vi "Protocol.Filter by Device Address.vi"(8 "error in":errorcluster, 10 "CAN Frame":T5 {"payload" format="%x"; "timestamp" format="%<%.7X\n%x>T"; "type" items=["CAN Data"=0, "CAN Remote"=1, "CAN Bus Error"=2, "CAN 2.0 Data"=8, "CAN FD Data"=16, "CAN FD+BRS Data"=24, "J1939 Data"=192, "Delay"=224, "Log Trigger"=225, "Start Trigger"=226]; "identifier" format="%x"}, 11 "J1939 Cluster":T2) -> (0 "error out":errorcluster, 1 "Pass Through":bool, 3 "State":T1=enum."ACL")   [LabVIEW 2023, in "J1939 Addon Engine.lvlib"]
uses:
  J1939 Addon Engine.lvlib
  <vilib>/xnet/xnet.llb/XNET Frame CAN.ctl
  <vilib>/xnet/xnet.llb/XNET Frame Type CAN.ctl
  Types/Protocol.Refs.ctl
  Support Libraries/J1939 Utilities/Types/CAN Outgoing Message Cluster.ctl
  Types/Protocol.RQST Lookup Table Reference.ctl
  Types/Protocol.Address Table Reference.ctl
  Support Libraries/J1939 Utilities/Types/Message Types.ctl
  Support Libraries/J1939 Utilities/J1939 Utilities.lvlib
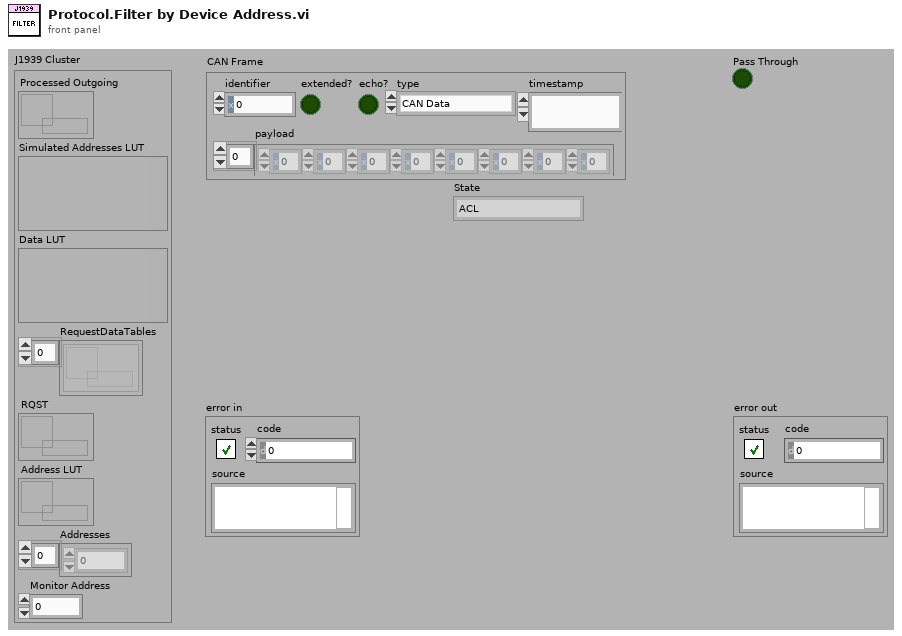
[diagram p1: front panel]
types:
  T1 = typedef "J1939 Utilities.lvlib/Message Types.ctl" = enum8{"PDU 1", "RQST2", "XFER", "ACKM", "RQST", "TP.DT - RTS/CTS", "TP.DT - BAM", "TP.CM - RTS", "TP.CM - CTS", "TP.CM - EndofMsgACK", "TP.CM - BAM", "TP.CM - Abort", "TP.CM - Error", "ACL", "Proprietary A", "PDU 2", "Proprietary B", "Error"}
  T2 = typedef "J1939 Addon Engine.lvlib/Protocol.Refs.ctl" = cluster{"Processed Outgoing":refnum<queue>, "Simulated Addresses LUT":variant, "Data LUT":variant, "RequestDataTables":refnum<k33>[], "RQST":T3, "Address LUT":T4, "Addresses":u8[], "Monitor Address":u8}
  T3 = typedef "J1939 Addon Engine.lvlib/Protocol.RQST Lookup Table Reference.ctl" = refnum<data-value>
  T4 = typedef "J1939 Addon Engine.lvlib/Protocol.Address Table Reference.ctl" = refnum<data-value>
  T5 = typedef "XNET Frame CAN.ctl" = cluster{"timestamp":timestamp, "payload":u8[], "identifier":u32, "type":T6, "extended?":bool, "echo?":bool}
  T6 = typedef "XNET Frame Type CAN.ctl" = u8
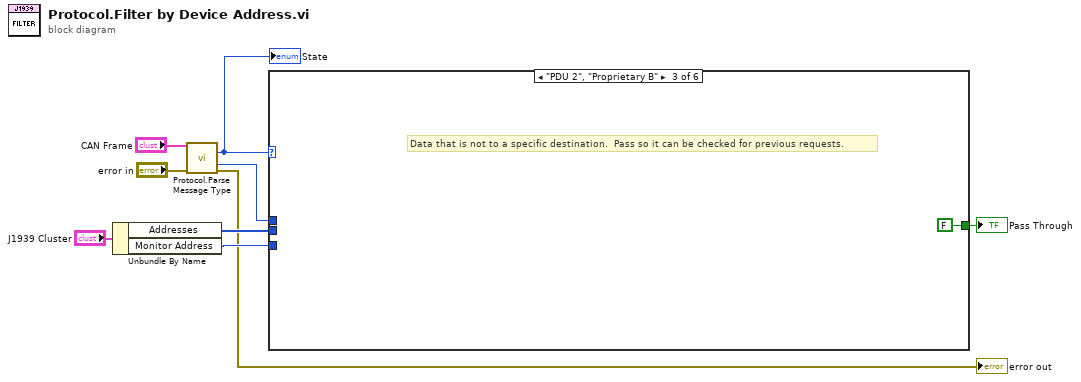
[diagram p0: block diagram]
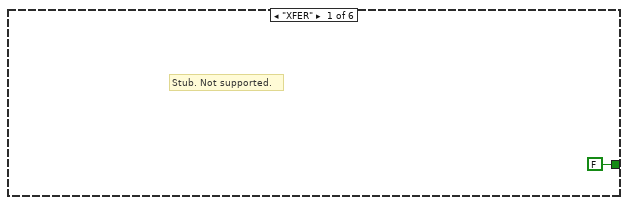
[diagram p2: hidden frame]
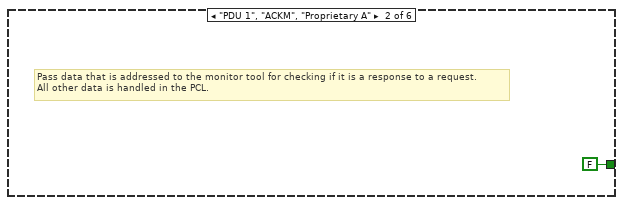
[diagram p3: hidden frame]
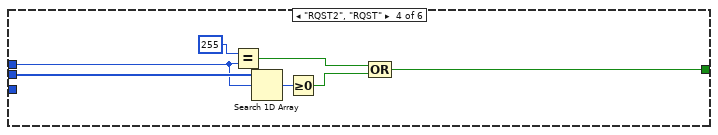
[diagram p4: hidden frame]
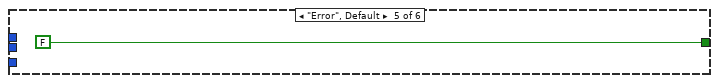
[diagram p5: hidden frame]
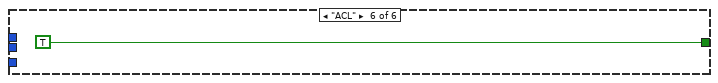
[diagram p6: hidden frame]
diagram:
  n1 = Unbundle By Name("J1939 Cluster") -> ("Addresses"=w3:u8[], "Monitor Address"=w2:u8)
  n2 = call "Protocol.Parse Message Type.vi"("CAN frame"="CAN Frame", "error in"="error in") -> ("State"=w9:T1, "PDU S"=w8:u8, "error out"=→"error out":errorcluster)  [unwired: 11 out]
  "State" <- w9
  n3 = case shown="\"PDU 2\", \"Proprietary B\"" w9 {
    tunnel: w3 -> [_ _ _ w15 _ _]
    tunnel: w8 -> [_ _ _ w14 _ _]
    tunnel: [FALSE FALSE FALSE w17 FALSE TRUE] -> w7
    tunnel: w2 -> [_ _ _ _ _ _]
    frame "XFER" {
      # "Stub. Not supported."
    }
    frame "PDU 1", "ACKM", "Proprietary A" {
      # "Pass data that is addressed to the monitor tool for checking if it is a response to a request.\nAll other data is handled in the PCL."
    }
    frame "PDU 2", "Proprietary B" {
      # "Data that is not to a specific destination.  Pass so it can be checked for previous requests."
    }
    frame "RQST2", "RQST" {
      n4 = Equal?(x=u8 255 ("y"), y=w14) -> (x = y?=w18:bool)
      n5 = Search 1D Array(1D array=w15, element=w14) -> (index of element=w16:i32)  [unwired: 1 in]
      n6 = Greater Or Equal To 0?(x=w16) -> (x >= 0?=w13:bool)
      n7 = Compound Arithmetic op=OR(w18, w13) -> (w17:bool)
    }
    frame "Error", Default {
    }
    frame "ACL" {
    }
  }
  "Pass Through" <- w7
